vi "destring_notifier_values.vi"(11 "input cluster 2":T1) -> (2 "Array 2":string[](array[string]), 3 "Array":string[](array[string]))   [LabVIEW 2013]
doc: "Takes a stringifed notifier and reads out the values"
uses:
  Data/TypeDefs/Log_Data.ctl
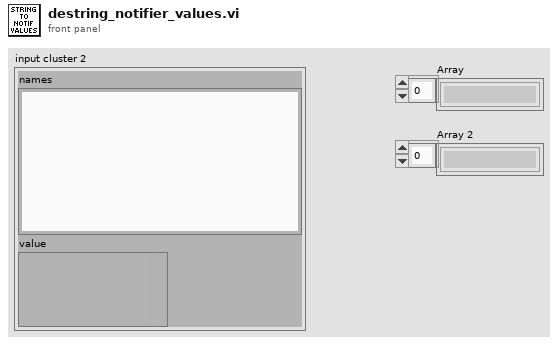
[diagram p1: front panel]
types:
  T1 = typedef "Log_Data.ctl" = cluster{"names":string, "value":variant}
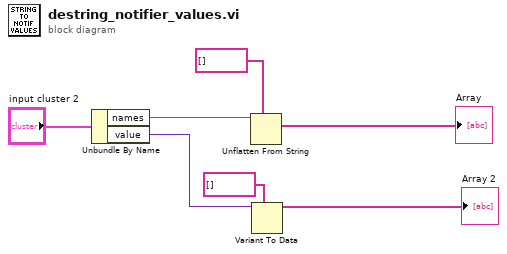
[diagram p0: block diagram]
diagram:
  n1 = Unbundle By Name("input cluster 2") -> ("names"=w5:string, "value"=w4:variant)
  n2 = Unflatten From String(type=string[] [] ("notifier names"), binary string=w5) -> (value=→"Array":string[])  [unwired: 3 in, 2 out]
  n3 = Variant To Data(type=string[] [], Variant=w4) -> (data=→"Array 2":string[])  [unwired: 1 in, 1 out]
